vi "Timing Estimation.vi"(1 "R":bool) -> (7 "dt (ms) out":u32)   [LabVIEW 2019, in "Timers.lvlib"]
uses:
  Timers.lvlib
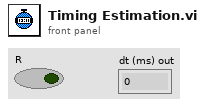
[diagram p1: front panel]
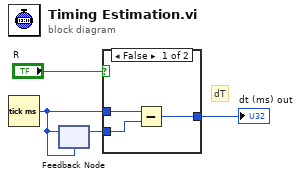
[diagram p0: block diagram]
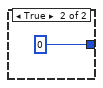
[diagram p2: hidden frame]
diagram:
  # "dT"
  n1 = Tick Count (ms)() -> (millisecond timer value=w2:u32)
  n2 = feedback #1(w2) -> (w3:u32)
  n3 = feedback-in #1(w2) -> ()
  n4 = case shown="False" "R" {
    tunnel: [w5 u32 0] -> w1
    tunnel: w3 -> [w6 _]
    tunnel: w2 -> [w7 _]
    frame False {
      n5 = Subtract(x=w7, y=w6) -> (x-y=w5:u32)
    }
    frame True {
    }
  }
  "dt (ms) out" <- w1
